vi "HAL camera info.vi"(2 "error in":errorcluster) -> (0 "error out":errorcluster, 1 "Andor Camera Properties":T1)   [LabVIEW 2015]
uses:
  HAL camera properties.ctl
  ATMCD32D.DLL
panel:
  out "VS Speeds (us/row)":sgl[](array[numeric])
  out "Number of VS Speeds":i32
  out "Preamp Gain Settings":sgl[](array[numeric])
  out "Number of Preamp Gains":i32
  out "Pixel V (um)":sgl
  out "Pixel H (um)":sgl
  out "Pixel Frequencies (MHz)\n(for each channel)":sgl[][](array[numeric])
  out "Number of HS Speeds\n(for each Channel)":i32[](array[numeric])
  out "Number of AD Channels":i32
  # "Camera:  Andor iXon/iXon Ultra"
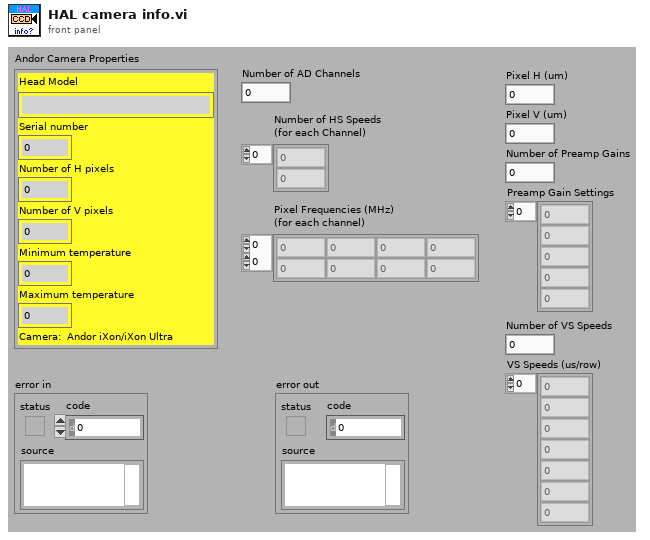
[diagram p1: front panel]
types:
  T1 = typedef "HAL camera properties.ctl" = cluster{"Head Model":string, "Serial number":i32, "Number of H pixels":i32, "Number of V pixels":i32, "Minimum temperature":i32, "Maximum temperature":i32}
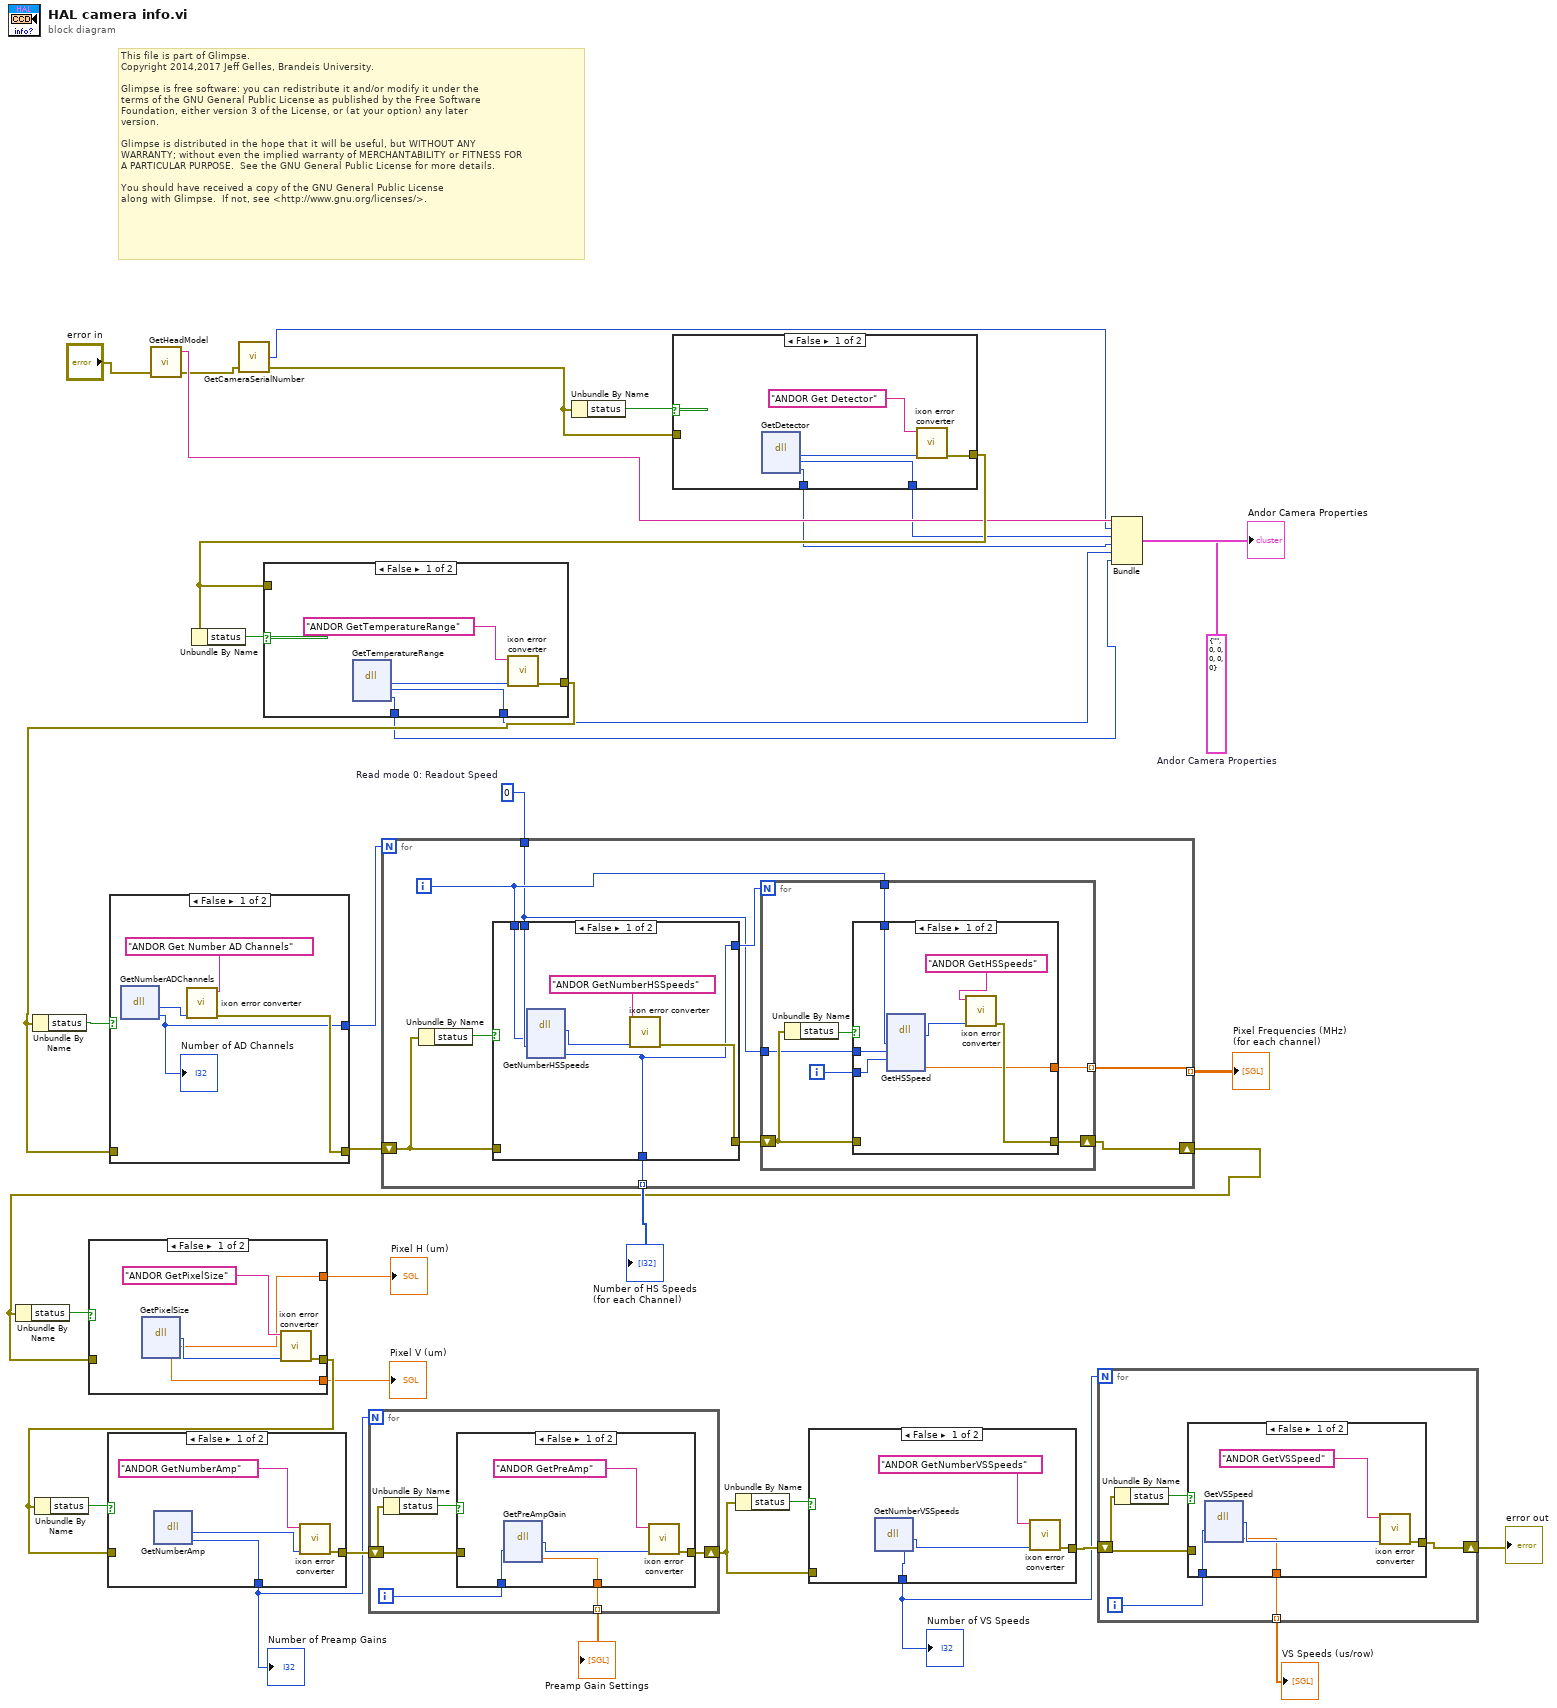
[diagram p0: block diagram]
diagram:
  w28 = 0  # Read mode 0: Readout Speed
  w33 = T1 {"Head Model"="", "Serial number"=0, "Number of H pixels"=0, "Number of V pixels"=0, "Minimum temperature"=0, "Maximum temperature"=0}  # Andor Camera Properties
  # "This file is part of Glimpse. \nCopyright 2014,2017 Jeff Gelles, Brandeis University.    \n\nGlimpse is free software: you can redistribute it and/or modify it under the \nterms of the GNU General Public License as published by the Free Software \nFoundation, either version 3 of the License, or (at your option) any later \nversion.\n\nGlimpse is distributed in the hope that it will be useful, but WITHOUT ANY \nWARRANTY; without even the implied warranty of MERCHANTABILITY or FITNESS FOR \nA PARTICULAR PURPOSE.  See the GNU General Public License for more details.\n\nYou should have received a copy of the GNU General Public License\nalong with Glimpse.  If not, see <http://www.gnu.org/licenses/>."
  n1 = call <userlib>:"GetHeadModel.vi"("error in (no error)"="error in") -> ("error out"=w7:errorcluster, "model"=w9:string)  [unwired: 2 in, 1 out]
  n2 = call <userlib>:"GetCameraSerialNumber.vi"("error in (no error)"=w7) -> ("error out"=w6:errorcluster, "number"=w1:i32)  [unwired: 2 in, 1 out]
  n3 = Unbundle By Name(w6) -> ("status"=w32:bool)
  n4 = case shown="False" w32 {
    tunnel: [w40 w42] -> w36
    tunnel: w6 -> [_ w42]
    tunnel: [w38 _] -> w3
    tunnel: [w37 _] -> w2
    frame False {
      n5 = dll-call lib="Atmcd32d.dll" fn="GetDetector" label="Get Detector"() -> (w39:u32, w37:i32, w38:i32)  [unwired: 3 in, 4 out]
      n6 = call "ixon error converter.vi"("Andor error code"=w39, "source"="ANDOR Get Detector") -> ("error out"=w40:errorcluster)  [unwired: 5 out]
    }
    frame True {
    }
  }
  n7 = Unbundle By Name(w36) -> ("status"=w35:bool)
  n8 = case shown="False" w35 {
    tunnel: [w46 w48] -> w31
    tunnel: [w44 _] -> w5
    tunnel: [w43 _] -> w4
    tunnel: w36 -> [_ w48]
    frame False {
      n9 = dll-call lib="Atmcd32d.dll" fn="GetTemperatureRange"() -> (w45:u32, w43:i32, w44:i32)  [unwired: 3 in, 4 out]
      n10 = call "ixon error converter.vi"("Andor error code"=w45, "source"="ANDOR GetTemperatureRange") -> ("error out"=w46:errorcluster)  [unwired: 5 out]
    }
    frame True {
    }
  }
  n11 = Unbundle By Name(w31) -> ("status"=w30:bool)
  n12 = case shown="False" w30 {
    tunnel: [w50 w53] -> w29
    tunnel: w31 -> [_ w53]
    tunnel: [w49 _] -> w10
    frame False {
      n13 = dll-call lib="Atmcd32d.dll" fn="GetNumberADChannels" label="Get Number AD Channels"() -> (w51:u32, w49:i32)  [unwired: 3 in, 3 out]
      "Number of AD Channels" <- w49
      n14 = call "ixon error converter.vi"("Andor error code"=w51, "source"="ANDOR Get Number AD Channels") -> ("error out"=w50:errorcluster)  [unwired: 5 out]
    }
    frame True {
    }
  }
  n15 = for {
    N: w10 -> [_]
    tunnel: [w61] -> w26 mode=indexing
    tunnel: w28 -> [w54]
    shift-right: [w56] -> w23
    shift-left: w29 -> [w59]
    tunnel: [w57] -> w27 mode=indexing
    i -> [w55]
    n16 = Unbundle By Name(w59) -> ("status"=w58:bool)
    n17 = case shown="False" w58 {
      tunnel: [w81 w84] -> w62
      tunnel: [w78 _] -> w60
      tunnel: w59 -> [_ w84]
      tunnel: w54 -> [w80 _]
      tunnel: w55 -> [w79 _]
      tunnel: [w78 _] -> w57
      frame False {
        n18 = dll-call lib="Atmcd32d.dll" fn="GetNumberHSSpeeds"(w79, w80) -> (w82:u32, w78:i32)  [unwired: 5 in, 3 out]
        n19 = call "ixon error converter.vi"("Andor error code"=w82, "source"="ANDOR GetNumberHSSpeeds") -> ("error out"=w81:errorcluster)  [unwired: 5 out]
      }
      frame True {
      }
    }
    n20 = for {
      N: w60 -> [_]
      shift-right: [w67] -> w56
      shift-left: w62 -> [w68]
      tunnel: [w66] -> w61 mode=indexing
      tunnel: w55 -> [w64]
      tunnel: w54 -> [w63]
      i -> [w65]
      n21 = Unbundle By Name(w68) -> ("status"=w69:bool)
      n22 = case shown="False" w69 {
        tunnel: w68 -> [_ w77]
        tunnel: [w74 w77] -> w67
        tunnel: [w73 _] -> w66
        tunnel: w65 -> [w72 _]
        tunnel: w64 -> [w71 _]
        tunnel: w63 -> [w70 _]
        frame False {
          n23 = dll-call lib="Atmcd32d.dll" fn="GetHSSpeed"(w71, w70, w72) -> (w75:u32, w73:sgl)  [unwired: 6 in, 3 out]
          n24 = call "ixon error converter.vi"("Andor error code"=w75, "source"="ANDOR GetHSSpeeds") -> ("error out"=w74:errorcluster)  [unwired: 5 out]
        }
        frame True {
        }
      }
    }
  }
  "Number of HS Speeds\n(for each Channel)" <- w27
  "Pixel Frequencies (MHz)\n(for each channel)" <- w26
  n25 = Unbundle By Name(w23) -> ("status"=w24:bool)
  n26 = case shown="False" w24 {
    tunnel: [w88 w90] -> w22
    tunnel: w23 -> [_ w90]
    tunnel: [w86 _] -> w20
    tunnel: [w85 _] -> w19
    frame False {
      n27 = dll-call lib="Atmcd32d.dll" fn="GetPixelSize"() -> (w87:u32, w85:sgl, w86:sgl)  [unwired: 3 in, 4 out]
      n28 = call "ixon error converter.vi"("Andor error code"=w87, "source"="ANDOR GetPixelSize") -> ("error out"=w88:errorcluster)  [unwired: 5 out]
    }
    frame True {
    }
  }
  "Pixel H (um)" <- w19
  "Pixel V (um)" <- w20
  n29 = Unbundle By Name(w22) -> ("status"=w25:bool)
  n30 = case shown="False" w25 {
    tunnel: [w93 w95] -> w21
    tunnel: w22 -> [_ w95]
    tunnel: [w92 _] -> w18
    frame False {
      n31 = dll-call lib="Atmcd32d.dll" fn="GetNumberAmp"() -> (w91:u32, w92:i32)  [unwired: 3 in, 3 out]
      n32 = call "ixon error converter.vi"("Andor error code"=w91, "source"="ANDOR GetNumberAmp") -> ("error out"=w93:errorcluster)  [unwired: 5 out]
    }
    frame True {
    }
  }
  "Number of Preamp Gains" <- w18
  n33 = for {
    N: w18 -> [_]
    tunnel: [w97] -> w17 mode=indexing
    shift-right: [w96] -> w16
    shift-left: w21 -> [w99]
    i -> [w98]
    n34 = Unbundle By Name(w99) -> ("status"=w100:bool)
    n35 = case shown="False" w100 {
      tunnel: [w104 w106] -> w96
      tunnel: w99 -> [_ w106]
      tunnel: w98 -> [w102 _]
      tunnel: [w101 _] -> w97
      frame False {
        n36 = dll-call lib="Atmcd32d.dll" fn="GetPreAmpGain" label="GetPreAmp"(w102) -> (w103:u32, w101:sgl)  [unwired: 4 in, 3 out]
        n37 = call "ixon error converter.vi"("Andor error code"=w103, "source"="ANDOR GetPreAmp") -> ("error out"=w104:errorcluster)  [unwired: 5 out]
      }
      frame True {
      }
    }
  }
  "Preamp Gain Settings" <- w17
  n38 = Unbundle By Name(w16) -> ("status"=w15:bool)
  n39 = case shown="False" w15 {
    tunnel: [w109 w111] -> w14
    tunnel: w16 -> [_ w111]
    tunnel: [w107 _] -> w13
    frame False {
      n40 = dll-call lib="Atmcd32d.dll" fn="GetNumberVSSpeeds"() -> (w108:u32, w107:i32)  [unwired: 3 in, 3 out]
      n41 = call "ixon error converter.vi"("Andor error code"=w108, "source"="ANDOR GetNumberVSSpeeds") -> ("error out"=w109:errorcluster)  [unwired: 5 out]
    }
    frame True {
    }
  }
  "Number of VS Speeds" <- w13
  n42 = for {
    N: w13 -> [_]
    shift-right: [w116] -> w11
    shift-left: w14 -> [w115]
    tunnel: [w113] -> w12 mode=indexing
    i -> [w114]
    n43 = Unbundle By Name(w115) -> ("status"=w112:bool)
    n44 = case shown="False" w112 {
      tunnel: [w120 w122] -> w116
      tunnel: w115 -> [_ w122]
      tunnel: w114 -> [w118 _]
      tunnel: [w117 _] -> w113
      frame False {
        n45 = dll-call lib="Atmcd32d.dll" fn="GetVSSpeed"(w118) -> (w119:u32, w117:sgl)  [unwired: 4 in, 3 out]
        n46 = call "ixon error converter.vi"("Andor error code"=w119, "source"="ANDOR GetVSSpeed") -> ("error out"=w120:errorcluster)  [unwired: 5 out]
      }
      frame True {
      }
    }
  }
  "error out" <- w11
  "VS Speeds (us/row)" <- w12
  n47 = Bundle(cluster=w33, "Head Model"=w9, "Serial number"=w1, "Number of H pixels"=w2, "Number of V pixels"=w3, "Minimum temperature"=w4, "Maximum temperature"=w5) -> (→"Andor Camera Properties":T1)
